vi "Cluster Item to Tree Item.vi"(7 "Action":T3=enum."Wire Properties", 10 "Index":i32, 11 "Cluster Element Data":T2) -> (2 "Disable":bool, 3 "Item":T1)   [LabVIEW 2023]
uses:
  controls/action enum.ctl
  Cluster Element Description.ctl
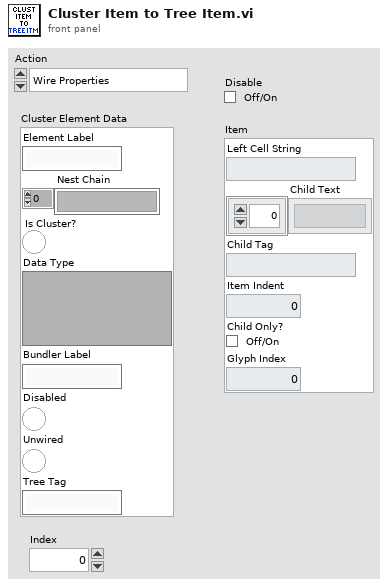
[diagram p1: front panel]
types:
  T1 = cluster{"Left Cell String":string, "Child Text":string[], "Child Tag":string, "Item Indent":i32, "Child Only?":bool, "Glyph Index":i32}
  T2 = typedef "Cluster Element Description.ctl" = cluster{"Element Label":string, "Nest Chain":string[], "Is Cluster?":bool, "Data Type":variant, "Bundler Label":string, "Disabled":bool, "Unwired":bool, "Tree Tag":string}
  T3 = typedef "action enum.ctl" = enum16{"[NONE]", "APP_SEPARATOR", "Wire Bundle", "Wire Unbundle", "Terminal Unbundle", "Terminal Bundle", "Bundler Move Up", "Bundler Move Down", "Bundler Insert", "Bundler Remove", "Bundler Remove Unwired", "Bundler Reorder", "In Place Insert", "In Place Remove", "In Place Remove Unwired", "In Place Reorder", "Wire Properties", "Wire Method", "Terminal Properties", "Terminal Method", "Property Move Up", "Property Move Down", "Properties Insert", "Properties Remove", "Properties Remove Unwired", "Properties Reorder", "Method Change", "Class For Constant", "Class For Control", "Class For Node", "Class Name to Clipboard"}
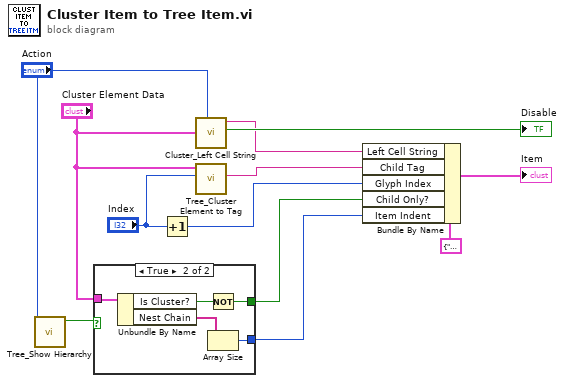
[diagram p0: block diagram]
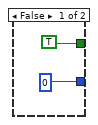
[diagram p2: hidden frame]
diagram:
  n1 = call "Tree_Show Hierarchy.vi"("Action"="Action") -> ("Show Heirarchy in Tree?"=w3:bool)  [unwired: 10 in]
  n2 = case shown="True" w3 {
    tunnel: "Cluster Element Data" -> [_ w16]
    tunnel: [TRUE w19] -> w8
    tunnel: [0 w17] -> w2
    frame False {
    }
    frame True {
      n3 = Unbundle By Name(w16) -> ("Is Cluster?"=w18:bool, "Nest Chain"=w15:string[])
      n4 = Not(x=w18) -> (.not. x?=w19:bool)
      n5 = Array Size(array=w15) -> (size(s)=w17:i32)
    }
  }
  n6 = Increment(x="Index") -> (x+1=w7:i32)
  n7 = call "Cluster_Left Cell String.vi"("Action"="Action", "Cluster Element Data"="Cluster Element Data") -> ("Disable"=→"Disable":bool, "Left Cell String"=w11:string)  [unwired: 8 in]
  n8 = call "Tree_Cluster Element to Tag.vi"("Index"="Index", "Cluster Element Data"="Cluster Element Data") -> ("Tree Tag Value"=w1:string)  [unwired: 8 in, 1 out]
  n9 = Bundle By Name(cluster=T1 {"Left Cell String"="", "Child Text"=[], "Child Tag"="", "Item Indent"=0, "Child Only?"=FALSE, "Glyph Index"=0} ("Item"), "Left Cell String"=w11, "Child Tag"=w1, "Glyph Index"=w7, "Child Only?"=w8, "Item Indent"=w2) -> (→"Item":T1)
